vi "PathPlanner_Path_ConstraintsForWaypointPos.vi"(9 "GlobalConstraints":T1={"MaxVelocityMps;"=0.0, "MaxAccelerationMpsSq;"=0.0, "MaxAngularVelRadPsEc;"=0.0, "MaxAngularAccRadPSecSq"=0.0, "Exists"=FALSE, "Unlimited"=FALSE, "NominalVoltageVolts"=12.0}, 10 "ConstraintsZones":T2[](array[typedef]), 11 "Pos":dbl) -> (3 "outPathPlannerPathConstraints":T1={"MaxVelocityMps;"=0.0, "MaxAccelerationMpsSq;"=0.0, "MaxAngularVelRadPsEc;"=0.0, "MaxAngularAccRadPSecSq"=0.0, "Exists"=FALSE, "Unlimited"=FALSE, "NominalVoltageVolts"=12.0})   [LabVIEW 2019, in "PathPlanner24.lvlib"]
doc: "Get the number of points in this path\n\nInputs: \n - Path - cluster - path definition data structure\n\nOutputs:\n - NumPoints - integer - Number of points in the path"
uses:
  PathPlanner24.lvlib
  TypeDef/PathPlannerPathConstraints.ctl
  TypeDef/PathPlannerConstraintsZone.ctl
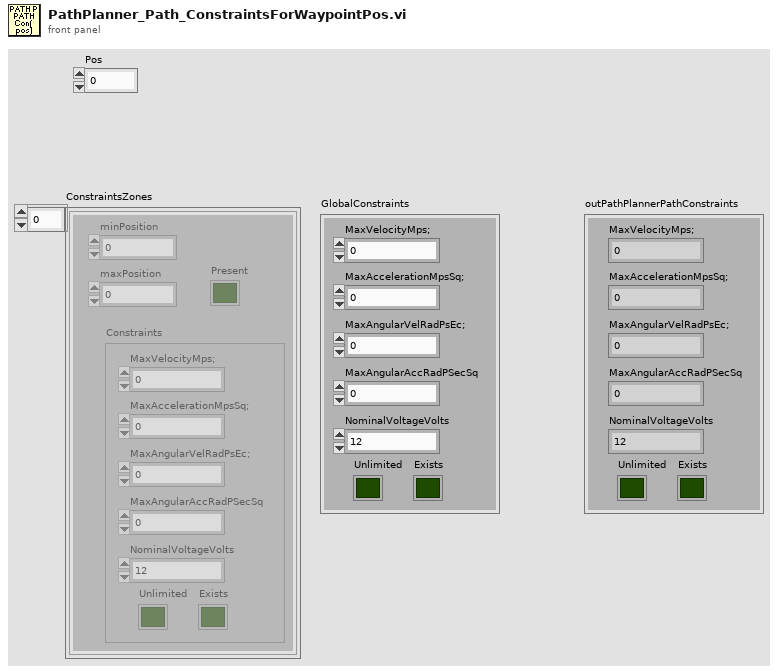
[diagram p1: front panel]
types:
  T1 = typedef "PathPlanner24.lvlib/PathPlannerPathConstraints.ctl" = cluster{"MaxVelocityMps;":dbl, "MaxAccelerationMpsSq;":dbl, "MaxAngularVelRadPsEc;":dbl, "MaxAngularAccRadPSecSq":dbl, "Exists":bool, "Unlimited":bool, "NominalVoltageVolts":dbl}
  T2 = typedef "PathPlanner24.lvlib/PathPlannerConstraintsZone.ctl" = cluster{"minPosition":dbl, "maxPosition":dbl, "Constraints":T1, "Present":bool}
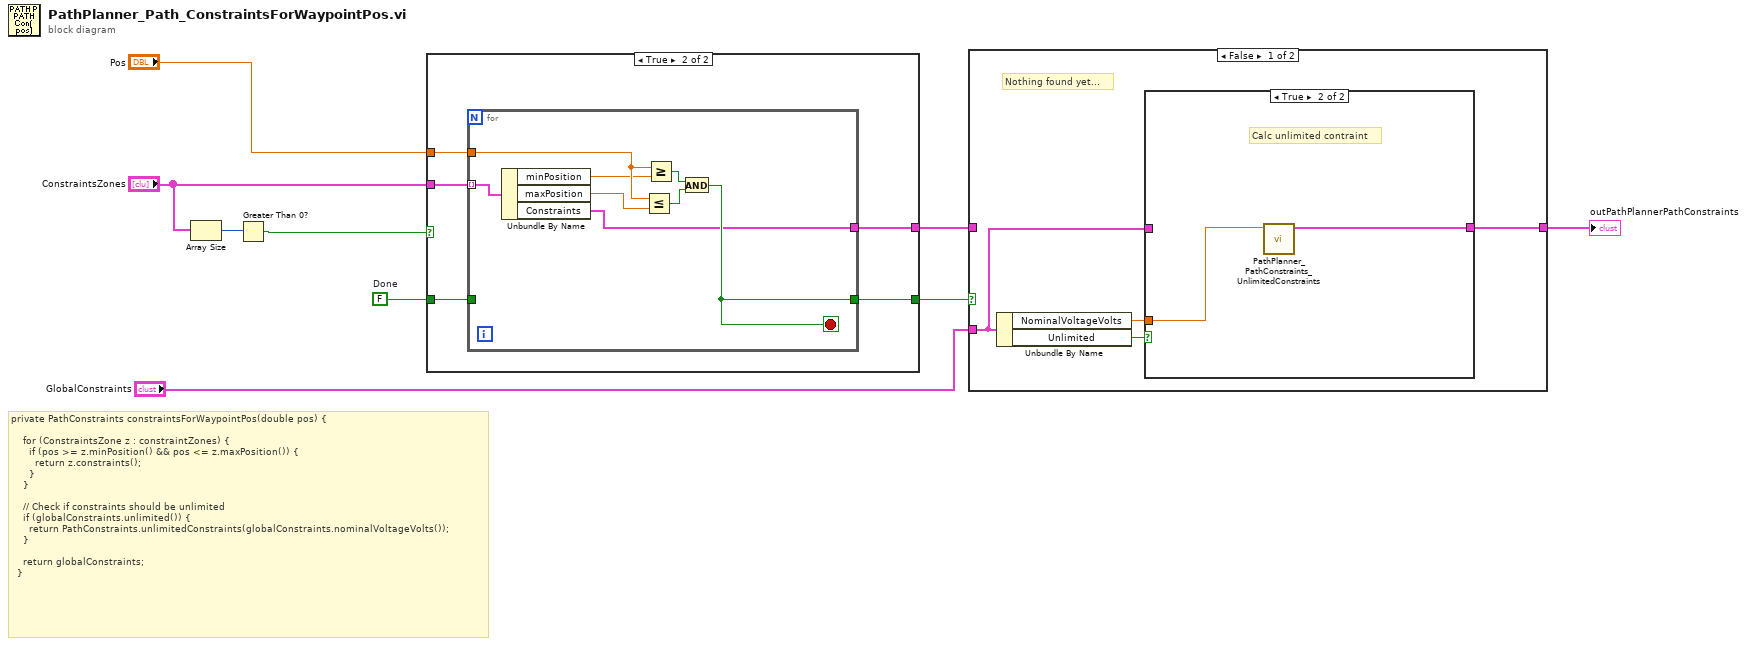
[diagram p0: block diagram]
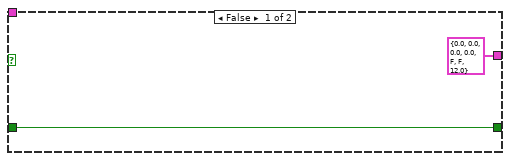
[diagram p4: hidden frame]
diagram:
  w7 = FALSE  # Done
  # "private PathConstraints constraintsForWaypointPos(double pos) {\n\n    for (ConstraintsZone z : constraintZones) {\n      if (pos >= z.minPosition() && pos <= z.maxPosition()) {\n        return z.constraints();\n      }\n    }\n\n    // Check if constraints should be unlimited\n    if (globalConstraints.unlimited()) {\n      return PathConstraints.unlimitedConstraints(globalConstraints.nominalVoltageVolts());\n    }\n\n    return globalConstraints;\n  }"
  n1 = Array Size(array="ConstraintsZones") -> (size(s)=w9:i32)
  n2 = Greater Than 0?(x=w9) -> (x > 0?=w8:bool)
  n3 = case shown="True" w8 {
    tunnel: w7 -> [w11 w16]
    tunnel: [w11 w12] -> w4
    tunnel: "ConstraintsZones" -> [_ w15]
    tunnel: "Pos" -> [_ w14]
    tunnel: [T1 {"MaxVelocityMps;"=0.0, "MaxAccelerationMpsSq;"=0.0, "MaxAngularVelRadPsEc;"=0.0, "MaxAngularAccRadPSecSq"=0.0, "Exists"=FALSE, "Unlimited"=FALSE, "NominalVoltageVolts"=12.0} ("Constraints") w13] -> w3
    frame False {
    }
    frame True {
      n4 = for {
        tunnel: w16 -> [_]
        tunnel: w15 -> [w19] mode=indexing
        tunnel: w14 -> [w24]
        tunnel: [w17] -> w13
        tunnel: [w18] -> w12
        stop <- w18 stop-if-true
        n5 = Unbundle By Name(w19) -> ("minPosition"=w23:dbl, "maxPosition"=w22:dbl, "Constraints"=w17:T1)
        n6 = Less Or Equal?(x=w24, y=w22) -> (x <= y?=w20:bool)
        n7 = Greater Or Equal?(x=w24, y=w23) -> (x >= y?=w21:bool)
        n8 = And(x=w21, y=w20) -> (x .and. y?=w18:bool)
      }
    }
  }
  n9 = case shown="False" w4 {
    tunnel: w3 -> [_ w32]
    tunnel: [w26 w32] -> w2
    tunnel: "GlobalConstraints" -> [w25 _]
    frame False {
      # "Nothing found yet..."
      n10 = Unbundle By Name(w25) -> ("NominalVoltageVolts"=w27:dbl, "Unlimited"=w28:bool)
      n11 = case shown="True" w28 {
        tunnel: w27 -> [_ w31]
        tunnel: [w29 w30] -> w26
        tunnel: w25 -> [w29 _]
        frame False {
          # "Use global constraints"
        }
        frame True {
          # "Calc unlimited contraint"
          n12 = call "PathPlanner_PathConstraints_UnlimitedConstraints.vi"("NominalVoltage"=w31) -> ("PathPlannerConstraints"=w30:T1)  [unwired: 10 in]
        }
      }
    }
    frame True {
      # "A constraint was found, use it..."
    }
  }
  "outPathPlannerPathConstraints" <- w2
